vi "Record User Facing.vi"(11 "JoystickDevRef":T1) -> ()   [LabVIEW 2016]
uses:
  <vilib>/Rock Robotics/WPI/Joystick/WPI_JoystickDevRef.ctl
  <vilib>/Rock Robotics/WPI/Joystick/WPI_JoystickDeviceEnum.ctl
  Robot Global Data.vi
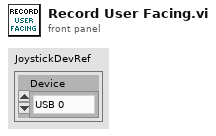
[diagram p1: front panel]
types:
  T1 = typedef "WPI_JoystickDevRef.ctl" = cluster{"Device":T2}
  T2 = typedef "WPI_JoystickDeviceEnum.ctl" = enum16{"USB 0", "USB 1", "USB 2", "USB 3", "USB 4", "USB 5"}
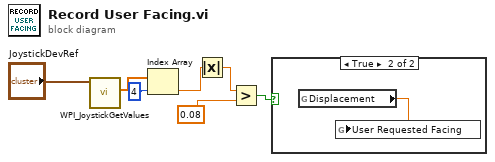
[diagram p0: block diagram]
diagram:
  n1 = call <vilib>:"WPI_JoystickGetValues.vi"("JoystickDevRef"="JoystickDevRef") -> ("Axes"=w7:dbl[])  [unwired: 6 in, 4 out]
  n2 = Index Array(array=w7, index=4) -> (element=w2:dbl)
  n3 = Absolute Value(x=w2) -> (abs(x)=w1:dbl)
  n4 = Greater?(x=w1, y=0.08) -> (0:w4:bool)
  n5 = case shown="True" w4 {
    frame False {
    }
    frame True {
      n6 = global read "Robot Global Data.vi" "Displacement"() -> (w8:dbl)
      n7 = global write "Robot Global Data.vi" "User Requested Facing"(w8) -> ()
    }
  }
